vi "test_Set-Get Protocol RSxxx.vi"(8 "error in (no error)":errorcluster, 11 "TestCase in":refnum<class "Instrument Addon Scripting API Custom Device Unit Tests.lvclass">) -> (0 "error out":errorcluster, 3 "TestCase out":refnum<class "Instrument Addon Scripting API Custom Device Unit Tests.lvclass">)   [LabVIEW 2019, in "Instrument Addon Scripting API Custom Device Unit Tests.lvclass"]
uses:
  Instrument Addon Scripting API Custom Device Unit Tests.lvclass
  Includes/Protocols.lvlibp/RS-xxx/RS-xxx.lvclass
  C:/Users/nitest/Desktop/Git/niveristand-instrument-addon-custom-device/Includes/Protocols.lvlibp/Protocol Parent/Protocol Parent.lvclass
  Includes/Protocols.lvlibp/AK RS-xxx/AK RS-xxx.lvclass
  Instrument Addon Scripting API Custom Device Unit Tests.lvclass/Instrument Addon Scripting API Custom Device Unit Tests.ctl
  Includes/Protocols.lvlibp/RS-xxx/Data Access/Write PortSettings.vi
  <vilib>/addons/_JKI Toolkits/VI Tester/TestCase.llb/TestCase.lvclass
  APIs/Scripting API/Instrument Addon Scripting API.lvlib
  C:/Program Files (x86)/National Instruments/LabVIEW 2019/vi.lib/addons/_JKI Toolkits/VI Tester/TestCase.llb/TestCase.lvclass
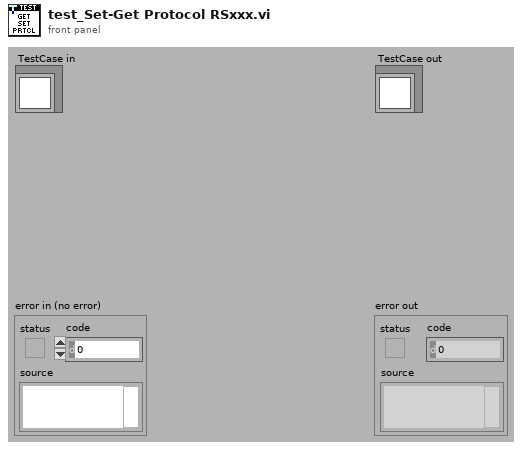
[diagram p1: front panel]
types:
  T1 = enum16{"NUL", "SOH", "STX", "ETX", "EOT", "ENQ", "ACK", "BEL", "BS", "HT", "LF", "VT", "FF", "CR", "SO", "SI", "DLE", "DC1", "DC2", "DC3", "DC4", "NAK", "SYN", "ETB", "CAN", "EM", "SUB", "ESC", "FS", "GS", "RS", "US", "SP", "!", "\"", "#", "$", "%", "&", "'", "(", ")", "*", "+", ",", "- (-)", ".", "/", "0", "1", "2", "3", "4", "5", "6", "7", "8", "9", ":", ";", "<", "=", ">", "?", "@", "A", "B", "C", "D", "E", "F", "G", "H", "I", "J", "K", "L", "M", "N", "O", "P", "Q", "R", "S", "T", "U", "V", "W", "X", "Y", "Z", "[", "\\", "]", "^", "_", "`", "a", "b", "c", "d", "e", "f", "g", "h", "i", "j", "k", "l", "m", "n", "o", "p", "q", "r", "s", "t", "u", "v", "w", "x", "y", "z", "{", "|", "}", "~"}
  T2 = cluster{"Port":string, "Baud Rate":u32, "Data Bits":u16, "Parity":enum16{"None", "Odd", "Even", "Mark", "Space"}, "Stop Bits":u16, "Flow Control":u16, "XON":enum16{"NUL", "SOH", "STX", "ETX", "EOT", "ENQ", "ACK", "BEL", "BS", "HT", "LF", "VT", "FF", "CR", "SO", "SI", "DLE", "DC1", "DC2", "DC3", "DC4", "NAK", "SYN", "ETB", "CAN", "EM", "SUB", "ESC", "FS", "GS", "RS", "US", "SP", "!", "\"", "#", "$", "%", "&", "'", "(", ")", "*", "+", ",", "- (-)", ".", "/", "0", "1", "2", "3", "4", "5", "6", "7", "8", "9", ":", ";", "<", "=", ">", "?", "@", "A", "B", "C", "D", "E", "F", "G", "H", "I", "J", "K", "L", "M", "N", "O", "P", "Q", "R", "S", "T", "U", "V", "W", "X", "Y", "Z", "[", "\\", "]", "^", "_", "`", "a", "b", "c", "d", "e", "f", "g", "h", "i", "j", "k", "l", "m", "n", "o", "p", "q", "r", "s", "t", "u", "v", "w", "x", "y", "z", "{", "|", "}", "~"}, "XOFF":enum16{"NUL", "SOH", "STX", "ETX", "EOT", "ENQ", "ACK", "BEL", "BS", "HT", "LF", "VT", "FF", "CR", "SO", "SI", "DLE", "DC1", "DC2", "DC3", "DC4", "NAK", "SYN", "ETB", "CAN", "EM", "SUB", "ESC", "FS", "GS", "RS", "US", "SP", "!", "\"", "#", "$", "%", "&", "'", "(", ")", "*", "+", ",", "- (-)", ".", "/", "0", "1", "2", "3", "4", "5", "6", "7", "8", "9", ":", ";", "<", "=", ">", "?", "@", "A", "B", "C", "D", "E", "F", "G", "H", "I", "J", "K", "L", "M", "N", "O", "P", "Q", "R", "S", "T", "U", "V", "W", "X", "Y", "Z", "[", "\\", "]", "^", "_", "`", "a", "b", "c", "d", "e", "f", "g", "h", "i", "j", "k", "l", "m", "n", "o", "p", "q", "r", "s", "t", "u", "v", "w", "x", "y", "z", "{", "|", "}", "~"}, "End Read on Termination Character":bool, "End Write on Termination Character":bool, "Termination Character":u8}
  T3 = typedef "Custom Device API.lvlib/Custom Device Item Ref.ctl" = u64
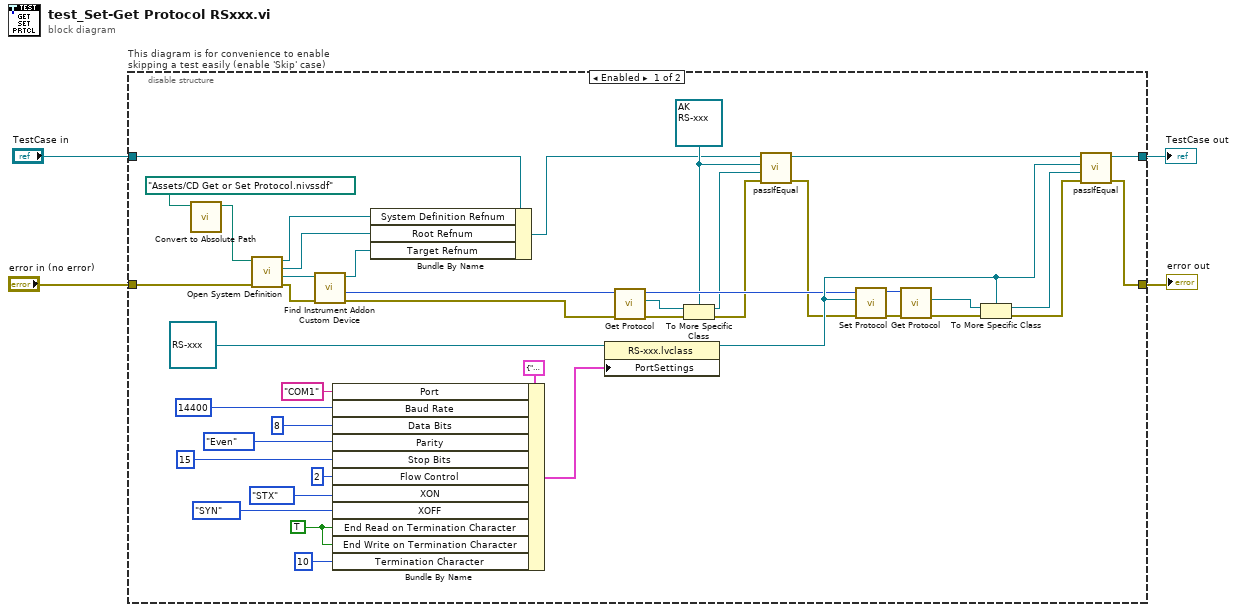
[diagram p0: block diagram]
diagram:
  n1 = disable-structure "This diagram is for convenience to enable skipping a test easily (enable 'Skip' case)" shown="Enabled" {
    disable-tunnel: "TestCase in" -> [w9 w50]
    disable-tunnel: [w36 w48] -> w1
    disable-tunnel: [w34 w49] -> w3
    disable-tunnel: "error in (no error)" -> [w46 w47]
    frame Enabled {
      w14 = refnum<class "AK RS-xxx.lvclass"> refnum ("reference out")
      w22 = TRUE ("End Read on Termination Character")
      n2 = call "Convert to Absolute Path.vi"("System Definition File"=path "Assets/CD Get or Set Protocol.nivssdf" ("SDF file")) -> ("Absolute Path"=w44:path)  [unwired: 10 in]
      n3 = call "Open System Definition.vi"("error in (no error)"=w46, "System Definition File"=w44) -> ("error out"=w43:errorcluster, "Target Refnum"=w42:refnum<k24>, "Root Refnum"=w7:refnum<k24>, "System Definition Refnum"=w8:refnum<k24>)  [unwired: 6 in]
      n4 = call "Find Instrument Addon Custom Device.vi"("error in"=w43, "target in"=w42) -> ("error out"=w19:errorcluster, "NodeID"=w20:u64, "target out"=w6:refnum<k24>)  [unwired: 7 in]
      n5 = Bundle By Name(cluster=T2 {"Port"="COM1", "Baud Rate"=9600, "Data Bits"=8, "Parity"=enum."None", "Stop Bits"=10, "Flow Control"=0, "XON"=enum."DC1", "XOFF"=enum."DC3", "End Read on Termination Character"=TRUE, "End Write on Termination Character"=TRUE, "Termination Character"=10} ("PortSettings"), "Port"="COM1", "Baud Rate"=u32 14400, "Data Bits"=u16 8, "Parity"=enum16{"None", "Odd", "Even", "Mark", "Space"}."Even", "Stop Bits"=u16 15, "Flow Control"=u16 2, "XON"=T1."STX", "XOFF"=T1."SYN", "End Read on Termination Character"=w22, "End Write on Termination Character"=w22, "Termination Character"=u8 10) -> (w31:T2)
      n6 = Bundle By Name(cluster=w9, "System Definition Refnum"=w8, "Root Refnum"=w7, "Target Refnum"=w6) -> (w5:refnum<class "Instrument Addon Scripting API Custom Device Unit Tests.lvclass">)
      n7 = property class="RS-xxx.lvclass"(reference=refnum<class "RS-xxx.lvclass"> refnum ("Protocols.lvlibp:RS-xxx.lvclass"), "PortSettings"=w31) -> (reference out=w17:refnum<class "RS-xxx.lvclass">)  [unwired: 1 in, 1 out]
      n8 = call "Get Protocol.vi"("error in (no error)"=w19, "instrument addon refnum in"=w20) -> ("error out"=w15:errorcluster, "protocol"=w18:refnum<class "Protocol Parent.lvclass">, "instrument addon refnum out"=w16:T3)  [unwired: 7 in]
      n9 = To More Specific Class(target class=w14, reference=w18, error in=w15) -> (specific class reference=w13:refnum<class "AK RS-xxx.lvclass">, error out=w12:errorcluster)
      n10 = call-dynamic "passIfEqual.vi"("error in (no error)"=w12, "y"=w13, "x"=w14, "TestCase in"=w5) -> ("error out"=w11:errorcluster, "TestCase out"=w10:refnum<class "Instrument Addon Scripting API Custom Device Unit Tests.lvclass">)  [unwired: 6 in]
      n11 = call "Set Protocol.vi"("error in (no error)"=w11, "protocol"=w17, "instrument addon refnum in"=w16) -> ("error out"=w40:errorcluster, "instrument addon refnum out"=w41:T3)  [unwired: 7 in]
      n12 = call "Get Protocol.vi"("error in (no error)"=w40, "instrument addon refnum in"=w41) -> ("error out"=w38:errorcluster, "protocol"=w39:refnum<class "Protocol Parent.lvclass">)  [unwired: 7 in, 1 out]
      n13 = To More Specific Class(target class=w17, reference=w39, error in=w38) -> (specific class reference=w35:refnum<class "RS-xxx.lvclass">, error out=w37:errorcluster)
      n14 = call-dynamic "passIfEqual.vi"("error in (no error)"=w37, "y"=w35, "x"=w17, "TestCase in"=w10) -> ("error out"=w34:errorcluster, "TestCase out"=w36:refnum<class "Instrument Addon Scripting API Custom Device Unit Tests.lvclass">)  [unwired: 6 in]
    }
    frame Disabled {
      # "skip test result while test is under development"
      n15 = call <vilib>:"skip.vi"("error in (no error)"=w47, "TestCase in"=w50) -> ("error out"=w49:errorcluster, "TestCase out"=w48:refnum<class "Instrument Addon Scripting API Custom Device Unit Tests.lvclass">)  [unwired: 8 in]
    }
  }
  "error out" <- w3
  "TestCase out" <- w1
